vi "newImageEvent.vi"(8 "error in (no error)":errorcluster, 9 "firstImage?":bool, 10 "Path":path, 11 "ImageStreamViewer in":refnum<class "ImageStreamViewer.lvclass">) -> (0 "error out":errorcluster, 3 "ImageStreamViewer out":refnum<class "ImageStreamViewer.lvclass">)   [LabVIEW 2011, in "Views.lvlib" / "Camera.lvlib" / "ImageStreamViewer.lvclass"]
uses:
  ImageStreamViewer.lvclass
  ImageStreamViewer.lvclass/ImageStreamViewer.ctl
panel:
  # "deal with a new image path arrival"
  # "clear ROI, add the path to the scroll bar, update the list of paths stored, display the image,\nupdate the image profiles, and update the image scale"
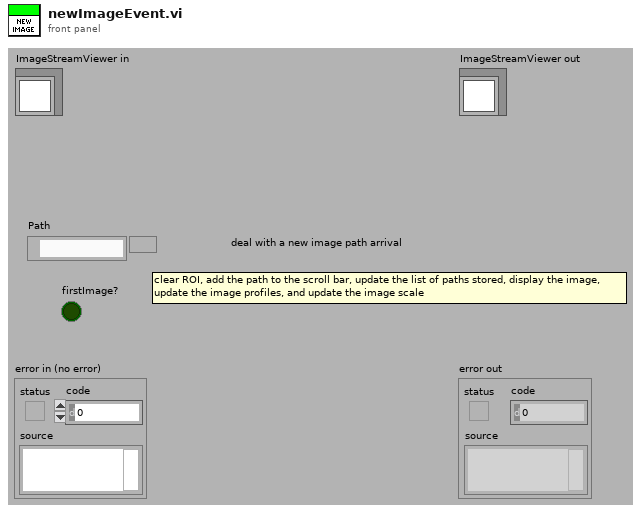
[diagram p1: front panel]
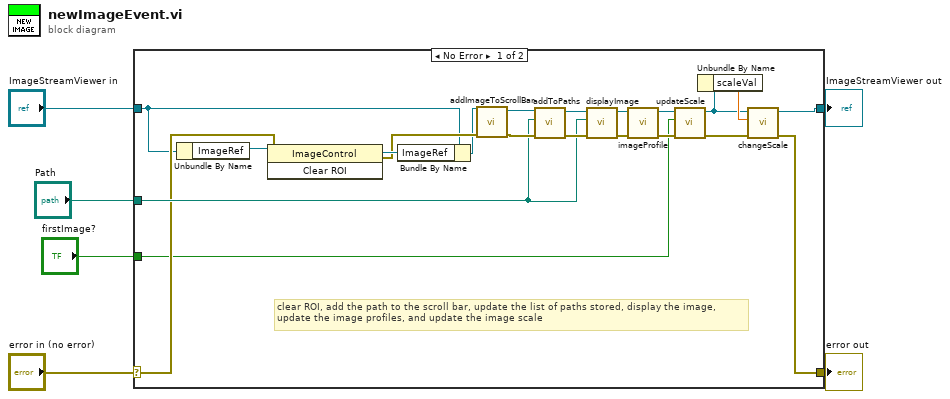
[diagram p0: block diagram]
diagram:
  n1 = case shown="No Error" "error in (no error)" {
    selector: "error in (no error)" -> [w18 w29]
    tunnel: [w13 w29] -> w5
    tunnel: [w14 w28] -> w3
    tunnel: "ImageStreamViewer in" -> [w16 w28]
    tunnel: "Path" -> [w23 _]
    tunnel: "firstImage?" -> [w7 _]
    frame No Error {
      # "clear ROI, add the path to the scroll bar, update the list of paths stored, display the image,\nupdate the image profiles, and update the image scale"
      n2 = Unbundle By Name(w16) -> ("ImageRef"=w20:refnum<vi>)
      n3 = invoke class="ImageControl" method="Clear ROI"(reference=w20, error in=w18) -> (reference out=w19:refnum<vi>, error out=w17:errorcluster)  [unwired: 1 in, 1 out]
      n4 = Bundle By Name(cluster=w16, "ImageRef"=w19) -> (w15:refnum<class "ImageStreamViewer.lvclass">)
      n5 = call "addImageToScrollBar.vi"("error in (no error)"=w17, "ImageStreamViewer in"=w15) -> ("error out"=w26:errorcluster, "ImageStreamViewer out"=w27:refnum<class "ImageStreamViewer.lvclass">)  [unwired: 8 in]
      n6 = call "addToPaths.vi"("error in (no error)"=w26, "Path"=w23, "ImageStreamViewer in"=w27) -> ("error out"=w24:errorcluster, "ImageStreamViewer out"=w25:refnum<class "ImageStreamViewer.lvclass">)  [unwired: 7 in]
      n7 = call "displayImage.vi"("error in (no error)"=w24, "Path"=w23, "ImageStreamViewer in"=w25) -> ("error out"=w21:errorcluster, "ImageStreamViewer out"=w22:refnum<class "ImageStreamViewer.lvclass">)  [unwired: 7 in]
      n8 = call "imageProfile.vi"("error in (no error)"=w21, "ImageStreamViewer in"=w22) -> ("error out"=w11:errorcluster, "ImageStreamViewer out"=w10:refnum<class "ImageStreamViewer.lvclass">)  [unwired: 8 in]
      n9 = call "updateScale.vi"("error in (no error)"=w11, "firstImage?"=w7, "ImageStreamViewer in"=w10) -> ("error out"=w8:errorcluster, "ImageStreamViewer out"=w9:refnum<class "ImageStreamViewer.lvclass">)  [unwired: 7 in]
      n10 = Unbundle By Name(w9) -> ("scaleVal"=w12:dbl)
      n11 = call "changeScale.vi"("error in (no error)"=w8, "newValue"=w12, "ImageStreamViewer in"=w9) -> ("error out"=w13:errorcluster, "ImageStreamViewer out"=w14:refnum<class "ImageStreamViewer.lvclass">)  [unwired: 7 in]
    }
    frame Error {
    }
  }
  "error out" <- w5
  "ImageStreamViewer out" <- w3
